vi "DataBuffer.vi"() -> ()   [LabVIEW 2014]
uses:
  <vilib>/Instr/_visa.llb/VISA Configure Serial Port (Instr).vi
panel:
  out "number":i32
  out "ResidualNum":string
  out "GatherRate":string
  out "Channel_state_a":string
  out "CURR?":string
  out "return count":u32
  out "Buffer Size":string
  out "State?":string
  in  "Keithley":refnum<visa-resource-name>
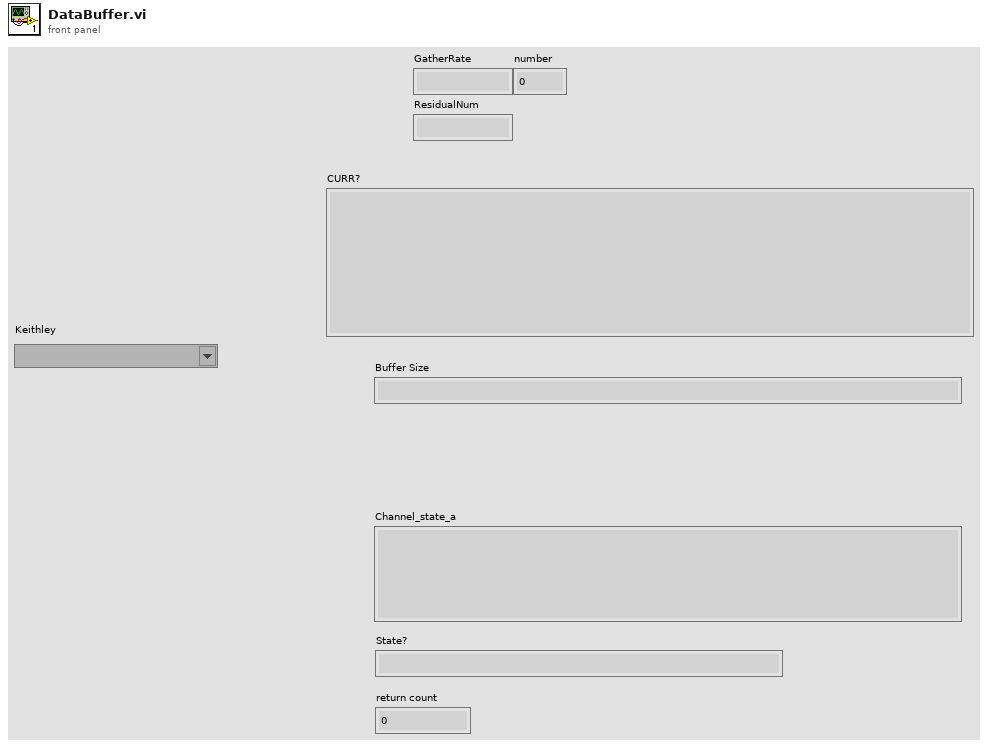
[diagram p1: front panel]
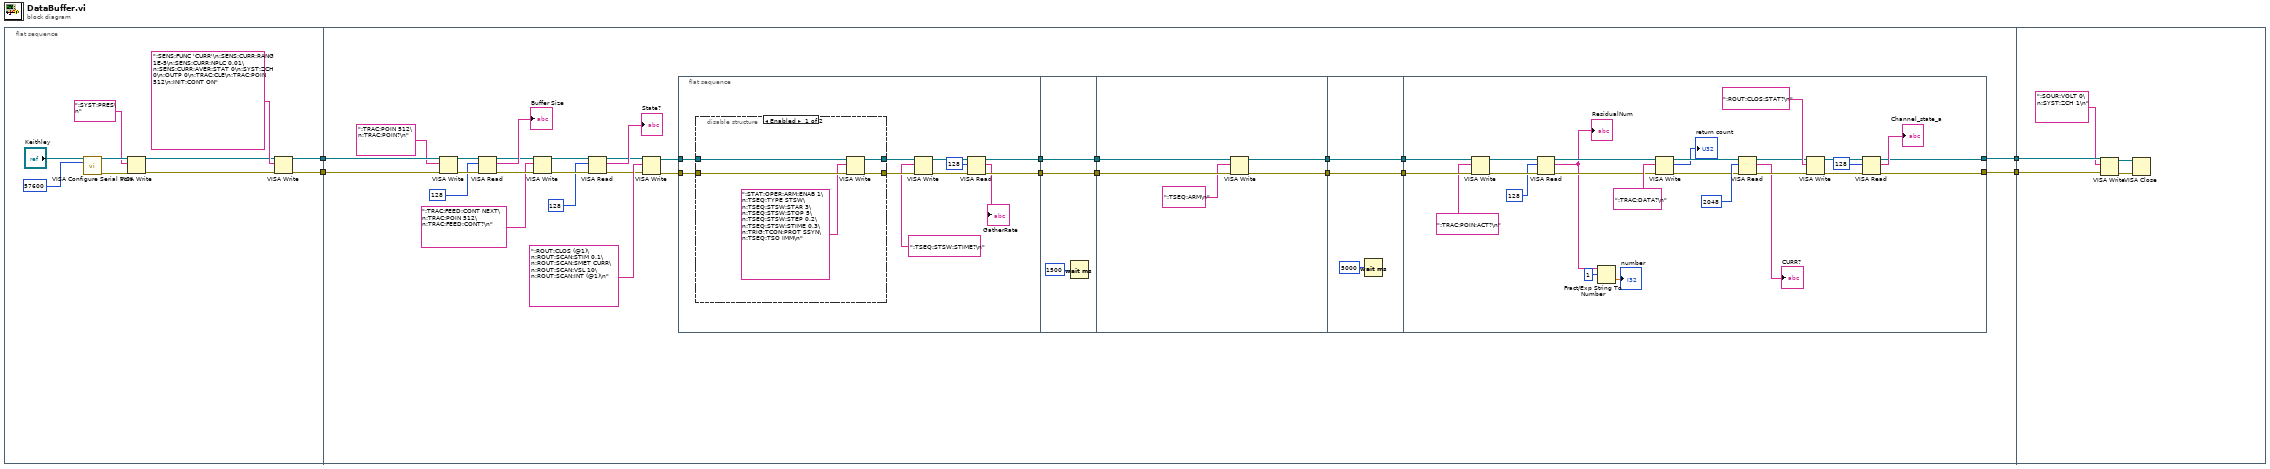
[diagram p0: block diagram]
diagram:
  n1 = flat-sequence {
    tunnel: [w6] -> w4
    tunnel: [w5] -> w3
    tunnel: w4 -> [w38]
    tunnel: w3 -> [w37]
    tunnel: [w42] -> w2
    tunnel: [w41] -> w1
    tunnel: w2 -> [w101]
    tunnel: w1 -> [w100]
    frame #0 {
      n2 = call-poly "VISA Configure Serial Port"("VISA resource name"="Keithley", "baud rate (9600)"=u32 57600) -> ("VISA resource name out"=w11:refnum<visa-resource-name>, "error out"=w10:errorcluster)  [unwired: 12 in]
      n3 = VISA Write(VISA resource name=w11, write buffer=":SYST:PRES\n", error in (no error)=w10) -> (VISA resource name out=w9:refnum<visa-resource-name>, error out=w8:errorcluster)  [unwired: 1 out]
      n4 = VISA Write(VISA resource name=w9, write buffer=":SENS:FUNC 'CURR'\n:SENS:CURR:RANG 1E-5\n:SENS:CURR:NPLC 0.01\n:SENS:CURR:AVER:STAT 0\n:SYST:ZCH 0\n:OUTP 0\n:TRAC:CLE\n:TRAC:POIN 512\n:INIT:CONT ON", error in (no error)=w8) -> (VISA resource name out=w6:refnum<visa-resource-name>, error out=w5:errorcluster)  [unwired: 1 out]
    }
    frame #1 {
      n5 = VISA Write(VISA resource name=w38, write buffer=":TRAC:POIN 512\n:TRAC:POIN?\n", error in (no error)=w37) -> (VISA resource name out=w35:refnum<visa-resource-name>, error out=w34:errorcluster)  [unwired: 1 out]
      n6 = VISA Read(VISA resource name=w35, byte count=u32 128, error in (no error)=w34) -> (VISA resource name out=w31:refnum<visa-resource-name>, read buffer=→"Buffer Size":string, error out=w30:errorcluster)  [unwired: 1 out]
      n7 = VISA Write(VISA resource name=w31, write buffer=":TRAC:FEED:CONT NEXT\n:TRAC:POIN 512\n:TRAC:FEED:CONT?\n", error in (no error)=w30) -> (VISA resource name out=w28:refnum<visa-resource-name>, error out=w27:errorcluster)  [unwired: 1 out]
      n8 = VISA Read(VISA resource name=w28, byte count=u32 128, error in (no error)=w27) -> (VISA resource name out=w24:refnum<visa-resource-name>, read buffer=→"State?":string, error out=w23:errorcluster)  [unwired: 1 out]
      n9 = VISA Write(VISA resource name=w24, write buffer=":ROUT:CLOS (@1)\n:ROUT:SCAN:STIM 0.1\n:ROUT:SCAN:SMET CURR\n:ROUT:SCAN:VSL 10\n:ROUT:SCAN:INT (@1)\n", error in (no error)=w23) -> (VISA resource name out=w21:refnum<visa-resource-name>, error out=w22:errorcluster)  [unwired: 1 out]
      n10 = flat-sequence {
        tunnel: w21 -> [w54]
        tunnel: w22 -> [w53]
        tunnel: [w46] -> w20
        tunnel: [w48] -> w19
        tunnel: w20 -> [w64]
        tunnel: [w64] -> w18
        tunnel: w19 -> [w63]
        tunnel: [w63] -> w16
        tunnel: w18 -> [w68]
        tunnel: [w66] -> w17
        tunnel: w16 -> [w69]
        tunnel: [w67] -> w15
        tunnel: [w71] -> w40
        tunnel: [w70] -> w39
        tunnel: w17 -> [w70]
        tunnel: w15 -> [w71]
        tunnel: [w85] -> w42
        tunnel: [w84] -> w41
        tunnel: w40 -> [w83]
        tunnel: w39 -> [w82]
        frame #0 {
          n11 = disable-structure shown="Enabled" {
            disable-tunnel: w54 -> [w59 w61]
            disable-tunnel: w53 -> [w58 w60]
            disable-tunnel: [w56 w61] -> w52
            disable-tunnel: [w55 w60] -> w51
            frame Enabled {
              n12 = VISA Write(VISA resource name=w59, write buffer=":STAT:OPER:ARM:ENAB 1\n:TSEQ:TYPE STSW\n:TSEQ:STSW:STAR 3\n:TSEQ:STSW:STOP 5\n:TSEQ:STSW:STEP 0.2\n:TSEQ:STSW:STIME 0.3\n:TRIG:TCON:PROT SSYN\n:TSEQ:TSO IMM\n", error in (no error)=w58) -> (VISA resource name out=w56:refnum<visa-resource-name>, error out=w55:errorcluster)  [unwired: 1 out]
            }
            frame Disabled {
            }
          }
          n13 = VISA Write(VISA resource name=w52, write buffer=":TSEQ:STSW:STIME?\n", error in (no error)=w51) -> (VISA resource name out=w49:refnum<visa-resource-name>, error out=w47:errorcluster)  [unwired: 1 out]
          n14 = VISA Read(VISA resource name=w49, byte count=u32 128, error in (no error)=w47) -> (VISA resource name out=w48:refnum<visa-resource-name>, read buffer=→"GatherRate":string, error out=w46:errorcluster)  [unwired: 1 out]
        }
        frame #1 {
          n15 = Wait (ms)(milliseconds to wait=u32 1500) -> ()  [unwired: 1 out]
        }
        frame #2 {
          n16 = VISA Write(VISA resource name=w69, write buffer=":TSEQ:ARM\n", error in (no error)=w68) -> (VISA resource name out=w67:refnum<visa-resource-name>, error out=w66:errorcluster)  [unwired: 1 out]
        }
        frame #3 {
          n17 = Wait (ms)(milliseconds to wait=u32 5000) -> ()  [unwired: 1 out]
        }
        frame #4 {
          n18 = VISA Write(VISA resource name=w83, write buffer=":TRAC:POIN:ACT?\n", error in (no error)=w82) -> (VISA resource name out=w81:refnum<visa-resource-name>, error out=w80:errorcluster)  [unwired: 1 out]
          n19 = VISA Read(VISA resource name=w81, byte count=u32 128, error in (no error)=w80) -> (VISA resource name out=w79:refnum<visa-resource-name>, read buffer=w75:string, error out=w78:errorcluster)  [unwired: 1 out]
          "ResidualNum" <- w75
          n20 = Fract/Exp String To Number(string=w75, offset=1) -> (number=→"number":dbl)  [unwired: 2 in, 1 out]
          n21 = VISA Write(VISA resource name=w79, write buffer=":TRAC:DATA?\n", error in (no error)=w78) -> (VISA resource name out=w89:refnum<visa-resource-name>, return count=→"return count":u32, error out=w88:errorcluster)
          n22 = VISA Read(VISA resource name=w89, byte count=u32 2048, error in (no error)=w88) -> (VISA resource name out=w93:refnum<visa-resource-name>, read buffer=→"CURR?":string, error out=w92:errorcluster)  [unwired: 1 out]
          n23 = VISA Write(VISA resource name=w93, write buffer=":ROUT:CLOS:STAT?\n", error in (no error)=w92) -> (VISA resource name out=w96:refnum<visa-resource-name>, error out=w97:errorcluster)  [unwired: 1 out]
          n24 = VISA Read(VISA resource name=w96, byte count=u32 128, error in (no error)=w97) -> (VISA resource name out=w85:refnum<visa-resource-name>, read buffer=→"Channel_state_a":string, error out=w84:errorcluster)  [unwired: 1 out]
        }
      }
    }
    frame #2 {
      n25 = VISA Write(VISA resource name=w101, write buffer=":SOUR:VOLT 0\n:SYST:ZCH 1\n", error in (no error)=w100) -> (VISA resource name out=w102:refnum<visa-resource-name>, error out=w103:errorcluster)  [unwired: 1 out]
      n26 = VISA Close(VISA resource name=w102, error in (no error)=w103) -> ()  [unwired: 1 out]
    }
  }
